vi "Hybrid car p.vi"   [LabVIEW 2016]
uses:
  <vilib>/NXT/Dual Mode Library/Waits/Wait_Num.vi
types:
  T1 = typedef "LVHSConnector.ctl" = refnum<class "BrickReference.lvclass">
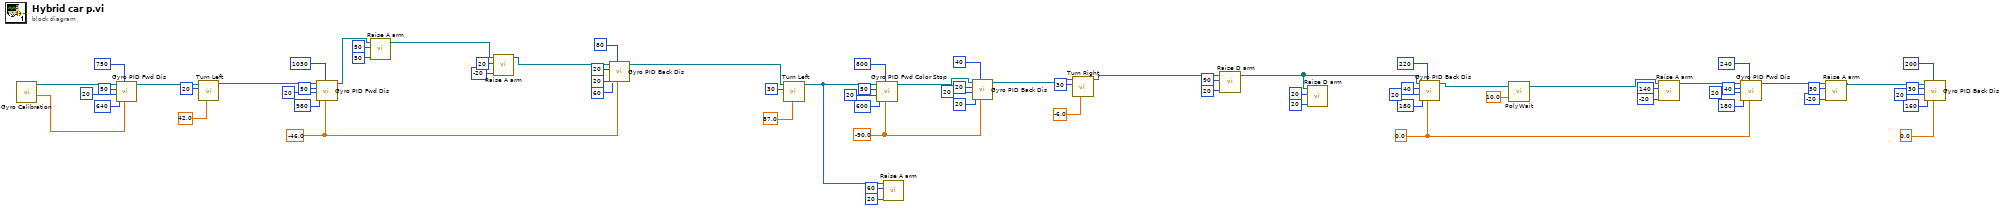
[diagram p0: block diagram]
diagram:
  w37 = sgl 0.0 ("Target angle")
  w33 = sgl -90.0 ("Target angle")
  w11 = sgl -46.0 ("Target angle")
  n1 = call "Gyro Calibration.vi"() -> ("Degrees"=w70:sgl, "NXT/EV3"=w75:T1)  [unwired: 7 in, 1 out]
  n2 = call "Gyro PID Fwd Dis.vi"("Target angle"=w70, "Threshold to stop"=750, "Threshold to slow"=640, "Min. speed"=20, "Max. speed"=50, "EV3 in"=w75) -> ("EV3 out"=w63:T1)  [unwired: 5 in]
  n3 = call "Turn Left.vi"("Turning angle"=sgl 42.0, "Motor B (right)"=i8 20, "EV3 in"=w63) -> ("EV3 out"=w62:T1)  [unwired: 8 in]
  n4 = call "Gyro PID Fwd Dis.vi"("Target angle"=w11, "Threshold to stop"=1030, "Threshold to slow"=980, "Min. speed"=20, "Max. speed"=50, "EV3 in"=w62) -> ("EV3 out"=w22:T1)  [unwired: 5 in]
  n5 = call "Raise A arm.vi"("Power"=i8 50, "Rotation"=50, "EV3 in"=w22) -> ("EV3 out"=w17:T1)  [unwired: 8 in]
  n6 = call "Raise A arm.vi"("Power"=i8 -20, "Rotation"=20, "EV3 in"=w17) -> ("EV3 out"=w16:T1)  [unwired: 8 in]
  n7 = call "Gyro PID Back Dis.vi"("Target angle"=w11, "Threshold to stop"=80, "Threshold to slow"=60, "Min. speed"=20, "Max. speed"=20, "EV3 in"=w16) -> ("EV3 out"=w15:T1)  [unwired: 5 in]
  n8 = call "Turn Left.vi"("Turning angle"=sgl 87.0, "Motor B (right)"=i8 30, "EV3 in"=w15) -> ("EV3 out"=w51:T1)  [unwired: 8 in]
  n9 = call "Gyro PID Fwd Color Stop.vi"("Target angle"=w33, "Threshold to Color"=800, "Threshold to slow"=600, "Min. speed"=20, "Max. speed"=50, "EV3 in"=w51) -> ("EV3 out"=w21:T1)  [unwired: 5 in]
  n10 = call "Raise A arm.vi"("Power"=i8 20, "Rotation"=60, "EV3 in"=w51) -> ()  [unwired: 8 in, 1 out]
  n11 = call "Gyro PID Back Dis.vi"("Target angle"=w33, "Threshold to stop"=40, "Threshold to slow"=20, "Min. speed"=20, "Max. speed"=20, "EV3 in"=w21) -> ("EV3 out"=w32:T1)  [unwired: 5 in]
  n12 = call "Turn Right.vi"("Turning angle"=sgl -6.0, "Motor B (right)"=i8 30, "EV3 in"=w32) -> ("EV3 out"=w8:T1)  [unwired: 8 in]
  n13 = call "Raise D arm.vi"("Power"=i8 20, "Rotation"=90, "EV3 in"=w8) -> ("EV3 out"=w2:T1)  [unwired: 8 in]
  n14 = call "Raise D arm.vi"("Power"=i8 20, "Rotation"=20, "EV3 in"=w2) -> ()  [unwired: 8 in, 1 out]
  n15 = call "Gyro PID Back Dis.vi"("Target angle"=w37, "Threshold to stop"=220, "Threshold to slow"=180, "Min. speed"=20, "Max. speed"=40, "EV3 in"=w2) -> ("EV3 out"=w5:T1)  [unwired: 5 in]
  n16 = call-poly <vilib>:"PolyWait.vi"("Time (1 sec)"=sgl 10.0, "NXT/EV3"=w5) -> ("NXT/EV3"=w4:T1)  [unwired: 2 in]
  n17 = call "Raise A arm.vi"("Power"=i8 -20, "Rotation"=140, "EV3 in"=w4) -> ("EV3 out"=w42:T1)  [unwired: 8 in]
  n18 = call "Gyro PID Fwd Dis.vi"("Target angle"=w37, "Threshold to stop"=240, "Threshold to slow"=180, "Min. speed"=20, "Max. speed"=40, "EV3 in"=w42) -> ("EV3 out"=w29:T1)  [unwired: 5 in]
  n19 = call "Raise A arm.vi"("Power"=i8 -20, "Rotation"=50, "EV3 in"=w29) -> ("EV3 out"=w23:T1)  [unwired: 8 in]
  n20 = call "Gyro PID Back Dis.vi"("Target angle"=sgl 0.0, "Threshold to stop"=200, "Threshold to slow"=160, "Min. speed"=20, "Max. speed"=30, "EV3 in"=w23) -> ()  [unwired: 5 in, 1 out]
